vi "test TCX read (installed 71).vi"() -> ()   [LabVIEW 2011] (continued)
nsion/v2\"><Watts>75</Watts></TPX></Extensions></Trackpoint><Trackpoint><Time>2008-03-03T23:08:00Z</Time><Position><LatitudeDegrees>35.861973</LatitudeDegrees><LongitudeDegrees>-78.884526</LongitudeDegrees></Position><AltitudeMeters>78.485</AltitudeMeters><DistanceMeters>12436.936</DistanceMeters><Cadence>73</Cadence><Extensions><TPX xmlns=\"http://www.garmin.com/xmlschemas/ActivityExtension/v2\"><Watts>74</Watts></TPX></Extensions></Trackpoint><Trackpoint><Time>2008-03-03T23:08:01Z</Time><Position><LatitudeDegrees>35.861915</LatitudeDegrees><LongitudeDegrees>-78.884579</LongitudeDegrees></Position><AltitudeMeters>77.523</AltitudeMeters><DistanceMeters>12444.917</DistanceMeters><Cadence>73</Cadence><Extensions><TPX xmlns=\"http://www.garmin.com/xmlschemas/ActivityExtension/v2\"><Watts>81</Watts></TPX></Extensions></Trackpoint><Trackpoint><Time>2008-03-03T23:08:02Z</Time><Position><LatitudeDegrees>35.861859</LatitudeDegrees><LongitudeDegrees>-78.884632</LongitudeDegrees></Position><AltitudeMeters>78.965</AltitudeMeters><DistanceMeters>12452.844</DistanceMeters><Cadence>73</Cadence><Extensions><TPX xmlns=\"http://www.garmin.com/xmlschemas/ActivityExtension/v2\"><Watts>81</Watts></TPX></Extensions></Trackpoint><Trackpoint><Time>2008-03-03T23:08:03Z</Time><Position><LatitudeDegrees>35.861803</LatitudeDegrees><LongitudeDegrees>-78.884687</LongitudeDegrees></Position><AltitudeMeters>78.004</AltitudeMeters><DistanceMeters>12460.762</DistanceMeters><Cadence>73</Cadence><Extensions><TPX xmlns=\"http://www.garmin.com/xmlschemas/ActivityExtension/v2\"><Watts>89</Watts></TPX></Extensions></Trackpoint><Trackpoint><Time>2008-03-03T23:08:04Z</Time><Position><LatitudeDegrees>35.861749</LatitudeDegrees><LongitudeDegrees>-78.884744</LongitudeDegrees></Position><AltitudeMeters>78.004</AltitudeMeters><DistanceMeters>12468.679</DistanceMeters><Cadence>72</Cadence><Extensions><TPX xmlns=\"http://www.garmin.com/xmlschemas/ActivityExtension/v2\"><Watts>91</Watts></TPX></Extensions></Trackpoint><Trackpoint><Time>2008-03-03T23:08:05Z</Time><Position><LatitudeDegrees>35.861695</LatitudeDegrees><LongitudeDegrees>-78.884802</LongitudeDegrees></Position><AltitudeMeters>78.485</AltitudeMeters><DistanceMeters>12476.672</DistanceMeters><Cadence>73</Cadence><Extensions><TPX xmlns=\"http://www.garmin.com/xmlschemas/ActivityExtension/v2\"><Watts>93</Watts></TPX></Extensions></Trackpoint><Trackpoint><Time>2008-03-03T23:08:06Z</Time><Position><LatitudeDegrees>35.861640</LatitudeDegrees><LongitudeDegrees>-78.884862</LongitudeDegrees></Position><AltitudeMeters>77.523</AltitudeMeters><DistanceMeters>12484.829</DistanceMeters><Cadence>75</Cadence><Extensions><TPX xmlns=\"http://www.garmin.com/xmlschemas/ActivityExtension/v2\"><Watts>87</Watts></TPX></Extensions></Trackpoint><Trackpoint><Time>2008-03-03T23:08:07Z</Time><Position><LatitudeDegrees>35.861583</LatitudeDegrees><LongitudeDegrees>-78.884922</LongitudeDegrees></Position><AltitudeMeters>77.043</AltitudeMeters><DistanceMeters>12493.188</DistanceMeters><Cadence>77</Cadence><Extensions><TPX xmlns=\"http://www.garmin.com/xmlschemas/ActivityExtension/v2\"><Watts>79</Watts></TPX></Extensions></Trackpoint><Trackpoint><Time>2008-03-03T23:08:08Z</Time><Position><LatitudeDegrees>35.861522</LatitudeDegrees><LongitudeDegrees>-78.884981</LongitudeDegrees></Position><AltitudeMeters>77.043</AltitudeMeters><DistanceMeters>12501.759</DistanceMeters><Cadence>77</Cadence><Extensions><TPX xmlns=\"http://www.garmin.com/xmlschemas/ActivityExtension/v2\"><Watts>79</Watts></TPX></Extensions></Trackpoint><Trackpoint><Time>2008-03-03T23:08:09Z</Time><Position><LatitudeDegrees>35.861459</LatitudeDegrees><LongitudeDegrees>-78.885040</LongitudeDegrees></Position><AltitudeMeters>77.043</AltitudeMeters><DistanceMeters>12510.541</DistanceMeters><Cadence>75</Cadence><Extensions><TPX xmlns=\"http://www.garmin.com/xmlschemas/ActivityExtension/v2\"><Watts>72</Watts></TPX></Extensions></Trackpoint><Trackpoint><Time>2008-03-03T23:08:10Z</Time><Position><LatitudeDegrees>35.861395</LatitudeDegrees><LongitudeDegrees>-78.885100</LongitudeDegrees></Position><AltitudeMeters>76.562</AltitudeMeters><DistanceMeters>12519.516</DistanceMeters><Cadence>67</Cadence><Extensions><TPX xmlns=\"http://www.garmin.com/xmlschemas/ActivityExtension/v2\"><Watts>71</Watts></TPX></Extensions></Trackpoint><Trackpoint><Time>2008-03-03T23:08:11Z</Time><Position><LatitudeDegrees>35.861330</LatitudeDegrees><LongitudeDegrees>-78.885161</LongitudeDegrees></Position><AltitudeMeters>76.081</AltitudeMeters><DistanceMeters>12528.636</DistanceMeters><Cadence>70</Cadence><Extensions><TPX xmlns=\"http://www.garmin.com/xmlschemas/ActivityExtension/v2\"><Watts>103</Watts></TPX></Extensions></Trackpoint><Trackpoint><Time>2008-03-03T23:08:12Z</Time><Position><LatitudeDegrees>35.861262</LatitudeDegrees><LongitudeDegrees>-78.885224</LongitudeDegrees></Position><AltitudeMeters>76.081</AltitudeMeters><DistanceMeters>12538.094</DistanceMeters><Cadence>70</Cadence><Extensions><TPX xmlns=\"http://www.garmin.com/xmlschemas/ActivityExtension/v2\"><Watts>102</Watts></TPX></Extensions></Trackpoint><Trackpoint><Time>2008-03-03T23:08:13Z</Time><Position><LatitudeDegrees>35.861193</LatitudeDegrees><LongitudeDegrees>-78.885289</LongitudeDegrees></Position><AltitudeMeters>76.081</AltitudeMeters><DistanceMeters>12547.728</DistanceMeters><Cadence>73</Cadence><Extensions><TPX xmlns=\"http://www.garmin.com/xmlschemas/ActivityExtension/v2\"><Watts>136</Watts></TPX></Extensions></Trackpoint><Trackpoint><Time>2008-03-03T23:08:14Z</Time><Position><LatitudeDegrees>35.861124</LatitudeDegrees><LongitudeDegrees>-78.885357</LongitudeDegrees></Position><AltitudeMeters>76.562</AltitudeMeters><DistanceMeters>12557.572</DistanceMeters><Cadence>74</Cadence><Extensions><TPX xmlns=\"http://www.garmin.com/xmlschemas/ActivityExtension/v2\"><Watts>141</Watts></TPX></Extensions></Trackpoint><Trackpoint><Time>2008-03-03T23:08:15Z</Time><Position><LatitudeDegrees>35.861052</LatitudeDegrees><LongitudeDegrees>-78.885425</LongitudeDegrees></Position><AltitudeMeters>75.601</AltitudeMeters><DistanceMeters>12567.610</DistanceMeters><Cadence>76</Cadence><Extensions><TPX xmlns=\"http://www.garmin.com/xmlschemas/ActivityExtension/v2\"><Watts>141</Watts></TPX></Extensions></Trackpoint><Trackpoint><Time>2008-03-03T23:08:16Z</Time><Position><LatitudeDegrees>35.860980</LatitudeDegrees><LongitudeDegrees>-78.885493</LongitudeDegrees></Position><AltitudeMeters>76.081</AltitudeMeters><DistanceMeters>12577.708</DistanceMeters><Cadence>76</Cadence><Extensions><TPX xmlns=\"http://www.garmin.com/xmlschemas/ActivityExtension/v2\"><Watts>124</Watts></TPX></Extensions></Trackpoint><Trackpoint><Time>2008-03-03T23:08:17Z</Time><Position><LatitudeDegrees>35.860907</LatitudeDegrees><LongitudeDegrees>-78.885559</LongitudeDegrees></Position><AltitudeMeters>75.601</AltitudeMeters><DistanceMeters>12587.827</DistanceMeters><Cadence>76</Cadence><Extensions><TPX xmlns=\"http://www.garmin.com/xmlschemas/ActivityExtension/v2\"><Watts>107</Watts></TPX></Extensions></Trackpoint><Trackpoint><Time>2008-03-03T23:08:18Z</Time><Position><LatitudeDegrees>35.860833</LatitudeDegrees><LongitudeDegrees>-78.885625</LongitudeDegrees></Position><AltitudeMeters>75.120</AltitudeMeters><DistanceMeters>12597.975</DistanceMeters><Cadence>77</Cadence><Extensions><TPX xmlns=\"http://www.garmin.com/xmlschemas/ActivityExtension/v2\"><Watts>106</Watts></TPX></Extensions></Trackpoint><Trackpoint><Time>2008-03-03T23:08:19Z</Time><Position><LatitudeDegrees>35.860758</LatitudeDegrees><LongitudeDegrees>-78.885691</LongitudeDegrees></Position><AltitudeMeters>76.081</AltitudeMeters><DistanceMeters>12608.146</DistanceMeters><Cadence>77</Cadence><Extensions><TPX xmlns=\"http://www.garmin.com/xmlschemas/ActivityExtension/v2\"><Watts>100</Watts></TPX></Extensions></Trackpoint><Trackpoint><Time>2008-03-03T23:08:20Z</Time><Position><LatitudeDegrees>35.860684</LatitudeDegrees><LongitudeDegrees>-78.885756</LongitudeDegrees></Position><AltitudeMeters>75.120</AltitudeMeters><DistanceMeters>12618.253</DistanceMeters><Cadence>76</Cadence><Extensions><TPX xmlns=\"http://www.garmin.com/xmlschemas/ActivityExtension/v2\"><Watts>97</Watts></TPX></Extensions></Trackpoint><Trackpoint><Time>2008-03-03T23:08:21Z</Time><Position><LatitudeDegrees>35.860610</LatitudeDegrees><LongitudeDegrees>-78.885821</LongitudeDegrees></Position><AltitudeMeters>74.640</AltitudeMeters><DistanceMeters>12628.325</DistanceMeters><Cadence>76</Cadence><Extensions><TPX xmlns=\"http://www.garmin.com/xmlschemas/ActivityExtension/v2\"><Watts>101</Watts></TPX></Extensions></Trackpoint><Trackpoint><Time>2008-03-03T23:08:22Z</Time><Position><LatitudeDegrees>35.860538</LatitudeDegrees><LongitudeDegrees>-78.885887</LongitudeDegrees></Position><AltitudeMeters>75.120</AltitudeMeters><DistanceMeters>12638.349</DistanceMeters><Cadence>76</Cadence><Extensions><TPX xmlns=\"http://www.garmin.com/xmlschemas/ActivityExtension/v2\"><Watts>94</Watts></TPX></Extensions></Trackpoint><Trackpoint><Time>2008-03-03T23:08:23Z</Time><Position><LatitudeDegrees>35.860466</LatitudeDegrees><LongitudeDegrees>-78.885953</LongitudeDegrees></Position><AltitudeMeters>74.640</AltitudeMeters><DistanceMeters>12648.291</DistanceMeters><Cadence>75</Cadence><Extensions><TPX xmlns=\"http://www.garmin.com/xmlschemas/ActivityExtension/v2\"><Watts>98</Watts></TPX></Extensions></Trackpoint><Trackpoint><Time>2008-03-03T23:08:24Z</Time><Position><LatitudeDegrees>35.860393</LatitudeDegrees><LongitudeDegrees>-78.886017</LongitudeDegrees></Position><AltitudeMeters>74.640</AltitudeMeters><DistanceMeters>12658.178</DistanceMeters><Cadence>75</Cadence><Extensions><TPX xmlns=\"http://www.garmin.com/xmlschemas/ActivityExtension/v2\"><Watts>92</Watts></TPX></Extensions></Trackpoint><Trackpoint><Time>2008-03-03T23:08:25Z</Time><Position><LatitudeDegrees>35.860320</LatitudeDegrees><LongitudeDegrees>-78.886080</LongitudeDegrees></Position><AltitudeMeters>74.159</AltitudeMeters><DistanceMeters>12668.053</DistanceMeters><Cadence>74</Cadence><Extensions><TPX xmlns=\"http://www.garmin.com/xmlschemas/ActivityExtension/v2\"><Watts>62</Watts></TPX></Extensions></Trackpoint><Trackpoint><Time>2008-03-03T23:08:26Z</Time><Position><LatitudeDegrees>35.860248</LatitudeDegrees><LongitudeDegrees>-78.886143</LongitudeDegrees></Position><AltitudeMeters>74.159</AltitudeMeters><DistanceMeters>12677.914</DistanceMeters><Cadence>74</Cadence><Extensions><TPX xmlns=\"http://www.garmin.com/xmlschemas/ActivityExtension/v2\"><Watts>62</Watts></TPX></Extensions></Trackpoint><Trackpoint><Time>2008-03-03T23:08:27Z</Time><Position><LatitudeDegrees>35.860178</LatitudeDegrees><LongitudeDegrees>-78.886208</LongitudeDegrees></Position><AltitudeMeters>74.159</AltitudeMeters><DistanceMeters>12687.683</DistanceMeters><Cadence>0</Cadence></Trackpoint><Trackpoint><Time>2008-03-03T23:08:28Z</Time><Position><LatitudeDegrees>35.860108</LatitudeDegrees><LongitudeDegrees>-78.886273</LongitudeDegrees></Position><AltitudeMeters>73.678</AltitudeMeters><DistanceMeters>12697.343</DistanceMeters><Cadence>0</Cadence></Trackpoint><Trackpoint><Time>2008-03-03T23:08:29Z</Time><Position><LatitudeDegrees>35.860044</LatitudeDegrees><LongitudeDegrees>-78.886338</LongitudeDegrees></Position><AltitudeMeters>73.198</AltitudeMeters><DistanceMeters>12706.586</DistanceMeters><Cadence>0</Cadence></Trackpoint><Trackpoint><Time>2008-03-03T23:08:30Z</Time><Position><LatitudeDegrees>35.859989</LatitudeDegrees><LongitudeDegrees>-78.886398</LongitudeDegrees></Position><AltitudeMeters>72.236</AltitudeMeters><DistanceMeters>12714.678</DistanceMeters><Cadence>12</Cadence></Trackpoint><Trackpoint><Time>2008-03-03T23:08:31Z</Time><Position><LatitudeDegrees>35.859945</LatitudeDegrees><LongitudeDegrees>-78.886452</LongitudeDegrees></Position><AltitudeMeters>72.236</AltitudeMeters><DistanceMeters>12721.393</DistanceMeters><Cadence>12</Cadence></Trackpoint><Trackpoint><Time>2008-03-03T23:08:32Z</Time><Position><LatitudeDegrees>35.859913</LatitudeDegrees><LongitudeDegrees>-78.886498</LongitudeDegrees></Position><AltitudeMeters>72.236</AltitudeMeters><DistanceMeters>12726.843</DistanceMeters><Cadence>0</Cadence></Trackpoint><Trackpoint><Time>2008-03-03T23:08:33Z</Time><Position><LatitudeDegrees>35.859889</LatitudeDegrees><LongitudeDegrees>-78.886536</LongitudeDegrees></Position><AltitudeMeters>72.236</AltitudeMeters><DistanceMeters>12731.098</DistanceMeters><Cadence>0</Cadence></Trackpoint><Trackpoint><Time>2008-03-03T23:08:34Z</Time><Position><LatitudeDegrees>35.859876</LatitudeDegrees><LongitudeDegrees>-78.886567</LongitudeDegrees></Position><AltitudeMeters>71.755</AltitudeMeters><DistanceMeters>12734.231</DistanceMeters><Cadence>18</Cadence></Trackpoint><Trackpoint><Time>2008-03-03T23:08:35Z</Time><Position><LatitudeDegrees>35.859867</LatitudeDegrees><LongitudeDegrees>-78.886602</LongitudeDegrees></Position><AltitudeMeters>71.755</AltitudeMeters><DistanceMeters>12737.604</DistanceMeters><Cadence>34</Cadence><Extensions><TPX xmlns=\"http://www.garmin.com/xmlschemas/ActivityExtension/v2\"><Watts>182</Watts></TPX></Extensions></Trackpoint><Trackpoint><Time>2008-03-03T23:08:36Z</Time><Position><LatitudeDegrees>35.859866</LatitudeDegrees><LongitudeDegrees>-78.886648</LongitudeDegrees></Position><AltitudeMeters>71.755</AltitudeMeters><DistanceMeters>12741.797</DistanceMeters><Cadence>34</Cadence><Extensions><TPX xmlns=\"http://www.garmin.com/xmlschemas/ActivityExtension/v2\"><Watts>179</Watts></TPX></Extensions></Trackpoint><Trackpoint><Time>2008-03-03T23:08:37Z</Time><Position><LatitudeDegrees>35.859876</LatitudeDegrees><LongitudeDegrees>-78.886705</LongitudeDegrees></Position><AltitudeMeters>71.755</AltitudeMeters><DistanceMeters>12747.175</DistanceMeters><Cadence>49</Cadence><Extensions><TPX xmlns=\"http://www.garmin.com/xmlschemas/ActivityExtension/v2\"><Watts>302</Watts></TPX></Extensions></Trackpoint><Trackpoint><Time>2008-03-03T23:08:38Z</Time><Position><LatitudeDegrees>35.859892</LatitudeDegrees><LongitudeDegrees>-78.886772</LongitudeDegrees></Position><AltitudeMeters>71.755</AltitudeMeters><DistanceMeters>12753.439</DistanceMeters><Cadence>58</Cadence><Extensions><TPX xmlns=\"http://www.garmin.com/xmlschemas/ActivityExtension/v2\"><Watts>428</Watts></TPX></Extensions></Trackpoint><Trackpoint><Time>2008-03-03T23:08:39Z</Time><Position><LatitudeDegrees>35.859909</LatitudeDegrees><LongitudeDegrees>-78.886846</LongitudeDegrees></Position><AltitudeMeters>71.755</AltitudeMeters><DistanceMeters>12760.476</DistanceMeters><Cadence>58</Cadence><Extensions><TPX xmlns=\"http://www.garmin.com/xmlschemas/ActivityExtension/v2\"><Watts>428</Watts></TPX></Extensions></Trackpoint><Trackpoint><Time>2008-03-03T23:08:40Z</Time><Position><LatitudeDegrees>35.859929</LatitudeDegrees><LongitudeDegrees>-78.886927</LongitudeDegrees></Position><AltitudeMeters>71.755</AltitudeMeters><DistanceMeters>12768.110</DistanceMeters><Cadence>74</Cadence><Extensions><TPX xmlns=\"http://www.garmin.com/xmlschemas/ActivityExtension/v2\"><Watts>465</Watts></TPX></Extensions></Trackpoint><Trackpoint><Time>2008-03-03T23:08:41Z</Time><Position><LatitudeDegrees>35.859949</LatitudeDegrees><LongitudeDegrees>-78.887013</LongitudeDegrees></Position><AltitudeMeters>72.236</AltitudeMeters><DistanceMeters>12776.246</DistanceMeters><Cadence>74</Cadence><Extensions><TPX xmlns=\"http://www.garmin.com/xmlschemas/ActivityExtension/v2\"><Watts>470</Watts></TPX></Extensions></Trackpoint><Trackpoint><Time>2008-03-03T23:08:42Z</Time><Position><LatitudeDegrees>35.859970</LatitudeDegrees><LongitudeDegrees>-78.887104</LongitudeDegrees></Position><AltitudeMeters>72.236</AltitudeMeters><DistanceMeters>12784.849</DistanceMeters><Cadence>79</Cadence><Extensions><TPX xmlns=\"http://www.garmin.com/xmlschemas/ActivityExtension/v2\"><Watts>395</Watts></TPX></Extensions></Trackpoint><Trackpoint><Time>2008-03-03T23:08:43Z</Time><Position><LatitudeDegrees>35.859993</LatitudeDegrees><LongitudeDegrees>-78.887199</LongitudeDegrees></Position><AltitudeMeters>72.236</AltitudeMeters><DistanceMeters>12793.792</DistanceMeters><Cadence>85</Cadence><Extensions><TPX xmlns=\"http://www.garmin.com/xmlschemas/ActivityExtension/v2\"><Watts>366</Watts></TPX></Extensions></Trackpoint><Trackpoint><Time>2008-03-03T23:08:44Z</Time><Position><LatitudeDegrees>35.860014</LatitudeDegrees><LongitudeDegrees>-78.887299</LongitudeDegrees></Position><AltitudeMeters>72.236</AltitudeMeters><DistanceMeters>12803.111</DistanceMeters><Cadence>87</Cadence><Extensions><TPX xmlns=\"http://www.garmin.com/xmlschemas/ActivityExtension/v2\"><Watts>420</Watts></TPX></Extensions></Trackpoint><Trackpoint><Time>2008-03-03T23:08:45Z</Time><Position><LatitudeDegrees>35.860035</LatitudeDegrees><LongitudeDegrees>-78.887402</LongitudeDegrees></Position><AltitudeMeters>72.717</AltitudeMeters><DistanceMeters>12812.741</DistanceMeters><Cadence>91</Cadence><Extensions><TPX xmlns=\"http://www.garmin.com/xmlschemas/ActivityExtension/v2\"><Watts>485</Watts></TPX></Extensions></Trackpoint><Trackpoint><Time>2008-03-03T23:08:46Z</Time><Position><LatitudeDegrees>35.860057</LatitudeDegrees><LongitudeDegrees>-78.887508</LongitudeDegrees></Position><AltitudeMeters>72.717</AltitudeMeters><DistanceMeters>12822.614</DistanceMeters><Cadence>92</Cadence><Extensions><TPX xmlns=\"http://www.garmin.com/xmlschemas/ActivityExtension/v2\"><Watts>483</Watts></TPX></Extensions></Trackpoint><Trackpoint><Time>2008-03-03T23:08:47Z</Time><Position><LatitudeDegrees>35.860078</LatitudeDegrees><LongitudeDegrees>-78.887616</LongitudeDegrees></Position><AltitudeMeters>73.678</AltitudeMeters><DistanceMeters>12832.634</DistanceMeters><Cadence>93</Cadence><Extensions><TPX xmlns=\"http://www.garmin.com/xmlschemas/ActivityExtension/v2\"><Watts>477</Watts></TPX></Extensions></Trackpoint><Trackpoint><Time>2008-03-03T23:08:48Z</Time><Position><LatitudeDegrees>35.860097</LatitudeDegrees><LongitudeDegrees>-78.887724</LongitudeDegrees></Position><AltitudeMeters>73.198</AltitudeMeters><DistanceMeters>12842.673</DistanceMeters><Cadence>93</Cadence><Extensions><TPX xmlns=\"http://www.garmin.com/xmlschemas/ActivityExtension/v2\"><Watts>388</Watts></TPX></Extensions></Trackpoint><Trackpoint><Time>2008-03-03T23:08:49Z</Time><Position><LatitudeDegrees>35.860116</LatitudeDegrees><LongitudeDegrees>-78.887833</LongitudeDegrees></Position><AltitudeMeters>73.198</AltitudeMeters><DistanceMeters>12852.671</DistanceMeters><Cadence>92</Cadence><Extensions><TPX xmlns=\"http://www.garmin.com/xmlschemas/ActivityExtension/v2\"><Watts>266</Watts></TPX></Extensions></Trackpoint><Trackpoint><Time>2008-03-03T23:08:50Z</Time><Position><LatitudeDegrees>35.860134</LatitudeDegrees><LongitudeDegrees>-78.887941</LongitudeDegrees></Position><AltitudeMeters>73.678</AltitudeMeters><DistanceMeters>12862.609</DistanceMeters><Cadence>91</Cadence><Extensions><TPX xmlns=\"http://www.garmin.com/xmlschemas/ActivityExtension/v2\"><Watts>169</Watts></TPX></Extensions></Trackpoint><Trackpoint><Time>2008-03-03T23:08:51Z</Time><Position><LatitudeDegrees>35.860150</LatitudeDegrees><LongitudeDegrees>-78.888048</LongitudeDegrees></Position><AltitudeMeters>73.678</AltitudeMeters><DistanceMeters>12872.501</DistanceMeters><Cadence>91</Cadence><Extensions><TPX xmlns=\"http://www.garmin.com/xmlschemas/ActivityExtension/v2\"><Watts>169</Watts></TPX></Extensions></Trackpoint><Trackpoint><Time>2008-03-03T23:08:52Z</Time><Position><LatitudeDegrees>35.860166</LatitudeDegrees><LongitudeDegrees>-78.888155</LongitudeDegrees></Position><AltitudeMeters>73.678</AltitudeMeters><DistanceMeters>12882.326</DistanceMeters><Cadence>90</Cadence><Extensions><TPX xmlns=\"http://www.garmin.com/xmlschemas/ActivityExtension/v2\"><Watts>150</Watts></TPX></Extensions></Trackpoint><Trackpoint><Time>2008-03-03T23:08:53Z</Time><Position><LatitudeDegrees>35.860180</LatitudeDegrees><LongitudeDegrees>-78.888263</LongitudeDegrees></Position><AltitudeMeters>73.198</AltitudeMeters><DistanceMeters>12892.139</DistanceMeters><Cadence>91</Cadence><Extensions><TPX xmlns=\"http://www.garmin.com/xmlschemas/ActivityExtension/v2\"><Watts>136</Watts></TPX></Extensions></Trackpoint><Trackpoint><Time>2008-03-03T23:08:54Z</Time><Position><LatitudeDegrees>35.860195</LatitudeDegrees><LongitudeDegrees>-78.888370</LongitudeDegrees></Position><AltitudeMeters>73.198</AltitudeMeters><DistanceMeters>12901.978</DistanceMeters><Cadence>80</Cadence><Extensions><TPX xmlns=\"http://www.garmin.com/xmlschemas/ActivityExtension/v2\"><Watts>121</Watts></TPX></Extensions></Trackpoint><Trackpoint><Time>2008-03-03T23:08:55Z</Time><Position><LatitudeDegrees>35.860208</LatitudeDegrees><LongitudeDegrees>-78.888479</LongitudeDegrees></Position><AltitudeMeters>73.678</AltitudeMeters><DistanceMeters>12911.919</DistanceMeters><Cadence>81</Cadence><Extensions><TPX xmlns=\"http://www.garmin.com/xmlschemas/ActivityExtension/v2\"><Watts>113</Watts></TPX></Extensions></Trackpoint><Trackpoint><Time>2008-03-03T23:08:56Z</Time><Position><LatitudeDegrees>35.860222</LatitudeDegrees><LongitudeDegrees>-78.888589</LongitudeDegrees></Position><AltitudeMeters>72.717</AltitudeMeters><DistanceMeters>12921.953</DistanceMeters><Cadence>82</Cadence><Extensions><TPX xmlns=\"http://www.garmin.com/xmlschemas/ActivityExtension/v2\"><Watts>115</Watts></TPX></Extensions></Trackpoint><Trackpoint><Time>2008-03-03T23:08:57Z</Time><Position><LatitudeDegrees>35.860233</LatitudeDegrees><LongitudeDegrees>-78.888701</LongitudeDegrees></Position><AltitudeMeters>72.717</AltitudeMeters><DistanceMeters>12932.187</DistanceMeters><Cadence>83</Cadence><Extensions><TPX xmlns=\"http://www.garmin.com/xmlschemas/ActivityExtension/v2\"><Watts>113</Watts></TPX></Extensions></Trackpoint><Trackpoint><Time>2008-03-03T23:08:58Z</Time><Position><LatitudeDegrees>35.860244</LatitudeDegrees><LongitudeDegrees>-78.888815</LongitudeDegrees></Position><AltitudeMeters>72.717</AltitudeMeters><DistanceMeters>12942.533</DistanceMeters><Cadence>86</Cadence><Extensions><TPX xmlns=\"http://www.garmin.com/xmlschemas/ActivityExtension/v2\"><Watts>81</Watts></TPX></Extensions></Trackpoint><Trackpoint><Time>2008-03-03T23:08:59Z</Time><Position><LatitudeDegrees>35.860255</LatitudeDegrees><LongitudeDegrees>-78.888931</LongitudeDegrees></Position><AltitudeMeters>72.236</AltitudeMeters><DistanceMeters>12953.332</DistanceMeters><Cadence>86</Cadence><Extensions><TPX xmlns=\"http://www.garmin.com/xmlschemas/ActivityExtension/v2\"><Watts>80</Watts></TPX></Extensions></Trackpoint><Trackpoint><Time>2008-03-03T23:09:00Z</Time><Position><LatitudeDegrees>35.860269</LatitudeDegrees><LongitudeDegrees>-78.889050</LongitudeDegrees></Position><AltitudeMeters>72.236</AltitudeMeters><DistanceMeters>12964.036</DistanceMeters><Cadence>89</Cadence><Extensions><TPX xmlns=\"http://www.garmin.com/xmlschemas/ActivityExtension/v2\"><Watts>84</Watts></TPX></Extensions></Trackpoint><Trackpoint><Time>2008-03-03T23:09:01Z</Time><Position><LatitudeDegrees>35.860285</LatitudeDegrees><LongitudeDegrees>-78.889171</LongitudeDegrees></Position><AltitudeMeters>71.755</AltitudeMeters><DistanceMeters>12975.059</DistanceMeters><Cadence>89</Cadence><Extensions><TPX xmlns=\"http://www.garmin.com/xmlschemas/ActivityExtension/v2\"><Watts>90</Watts></TPX></Extensions></Trackpoint><Trackpoint><Time>2008-03-03T23:09:02Z</Time><Position><LatitudeDegrees>35.860300</LatitudeDegrees><LongitudeDegrees>-78.889294</LongitudeDegrees></Position><AltitudeMeters>71.755</AltitudeMeters><DistanceMeters>12986.354</DistanceMeters><Cadence>87</Cadence><Extensions><TPX xmlns=\"http://www.garmin.com/xmlschemas/ActivityExtension/v2\"><Watts>115</Watts></TPX></Extensions></Trackpoint><Trackpoint><Time>2008-03-03T23:09:03Z</Time><Position><LatitudeDegrees>35.860315</LatitudeDegrees><LongitudeDegrees>-78.889421</LongitudeDegrees></Position><AltitudeMeters>71.275</AltitudeMeters><DistanceMeters>12997.958</DistanceMeters><Cadence>89</Cadence><Extensions><TPX xmlns=\"http://www.garmin.com/xmlschemas/ActivityExtension/v2\"><Watts>147</Watts></TPX></Extensions></Trackpoint><Trackpoint><Time>2008-03-03T23:09:04Z</Time><Position><LatitudeDegrees>35.860331</LatitudeDegrees><LongitudeDegrees>-78.889552</LongitudeDegrees></Position><AltitudeMeters>71.275</AltitudeMeters><DistanceMeters>13009.899</DistanceMeters><Cadence>92</Cadence><Extensions><TPX xmlns=\"http://www.garmin.com/xmlschemas/ActivityExtension/v2\"><Watts>145</Watts></TPX></Extensions></Trackpoint><Trackpoint><Time>2008-03-03T23:09:05Z</Time><Position><LatitudeDegrees>35.860348</LatitudeDegrees><LongitudeDegrees>-78.889685</LongitudeDegrees></Position><AltitudeMeters>70.794</AltitudeMeters><DistanceMeters>13022.080</DistanceMeters><Cadence>94</Cadence><Extensions><TPX xmlns=\"http://www.garmin.com/xmlschemas/ActivityExtension/v2\"><Watts>146</Watts></TPX></Extensions></Trackpoint><Trackpoint><Time>2008-03-03T23:09:06Z</Time><Position><LatitudeDegrees>35.860365</LatitudeDegrees><LongitudeDegrees>-78.889821</LongitudeDegrees></Position><AltitudeMeters>70.313</AltitudeMeters><DistanceMeters>13034.580</DistanceMeters><Cadence>94</Cadence><Extensions><TPX xmlns=\"http://www.garmin.com/xmlschemas/ActivityExtension/v2\"><Watts>145</Watts></TPX></Extensions></Trackpoint><Trackpoint><Time>2008-03-03T23:09:07Z</Time><Position><LatitudeDegrees>35.860383</LatitudeDegrees><LongitudeDegrees>-78.889961</LongitudeDegrees></Position><AltitudeMeters>70.313</AltitudeMeters><DistanceMeters>13047.376</DistanceMeters><Cadence>90</Cadence><Extensions><TPX xmlns=\"http://www.garmin.com/xmlschemas/ActivityExtension/v2\"><Watts>128</Watts></TPX></Extensions></Trackpoint><Trackpoint><Time>2008-03-03T23:09:08Z</Time><Position><LatitudeDegrees>35.860400</LatitudeDegrees><LongitudeDegrees>-78.890102</LongitudeDegrees></Position><AltitudeMeters>69.833</AltitudeMeters><DistanceMeters>13060.242</DistanceMeters><Cadence>92</Cadence><Extensions><TPX xmlns=\"http://www.garmin.com/xmlschemas/ActivityExtension/v2\"><Watts>125</Watts></TPX></Extensions></Trackpoint><Trackpoint><Time>2008-03-03T23:09:09Z</Time><Position><LatitudeDegrees>35.860418</LatitudeDegrees><LongitudeDegrees>-78.890245</LongitudeDegrees></Position><AltitudeMeters>69.833</AltitudeMeters><DistanceMeters>13073.274</DistanceMeters><Cadence>92</Cadence><Extensions><TPX xmlns=\"http://www.garmin.com/xmlschemas/ActivityExtension/v2\"><Watts>112</Watts></TPX></Extensions></Trackpoint><Trackpoint><Time>2008-03-03T23:09:10Z</Time><Position><LatitudeDegrees>35.860435</LatitudeDegrees><LongitudeDegrees>-78.890388</LongitudeDegrees></Position><AltitudeMeters>69.833</AltitudeMeters><DistanceMeters>13086.366</DistanceMeters><Cadence>92</Cadence><Extensions><TPX xmlns=\"http://www.garmin.com/xmlschemas/ActivityExtension/v2\"><Watts>95</Watts></TPX></Extensions></Trackpoint><Trackpoint><Time>2008-03-03T23:09:11Z</Time><Position><LatitudeDegrees>35.860454</LatitudeDegrees><LongitudeDegrees>-78.890529</LongitudeDegrees></Position><AltitudeMeters>69.352</AltitudeMeters><DistanceMeters>13099.340</DistanceMeters><Cadence>92</Cadence><Extensions><TPX xmlns=\"http://www.garmin.com/xmlschemas/ActivityExtension/v2\"><Watts>96</Watts></TPX></Extensions></Trackpoint><Trackpoint><Time>2008-03-03T23:09:12Z</Time><Position><LatitudeDegrees>35.860473</LatitudeDegrees><LongitudeDegrees>-78.890670</LongitudeDegrees></Position><AltitudeMeters>69.352</AltitudeMeters><DistanceMeters>13112.229</DistanceMeters><Cadence>90</Cadence><Extensions><TPX xmlns=\"http://www.garmin.com/xmlschemas/ActivityExtension/v2\"><Watts>85</Watts></TPX></Extensions></Trackpoint><Trackpoint><Time>2008-03-03T23:09:13Z</Time><Position><LatitudeDegrees>35.860491</LatitudeDegrees><LongitudeDegrees>-78.890808</LongitudeDegrees></Position><AltitudeMeters>68.872</AltitudeMeters><DistanceMeters>13124.790</DistanceMeters><Cadence>89</Cadence><Extensions><TPX xmlns=\"http://www.garmin.com/xmlschemas/ActivityExtension/v2\"><Watts>79</Watts></TPX></Extensions></Trackpoint><Trackpoint><Time>2008-03-03T23:09:14Z</Time><Position><LatitudeDegrees>35.860509</LatitudeDegrees><LongitudeDegrees>-78.890945</LongitudeDegrees></Position><AltitudeMeters>68.391</AltitudeMeters><DistanceMeters>13137.343</DistanceMeters><Cadence>88</Cadence><Extensions><TPX xmlns=\"http://www.garmin.com/xmlschemas/ActivityExtension/v2\"><Watts>80</Watts></TPX></Extensions></Trackpoint><Trackpoint><Time>2008-03-03T23:09:15Z</Time><Position><LatitudeDegrees>35.860528</LatitudeDegrees><LongitudeDegrees>-78.891081</LongitudeDegrees></Position><AltitudeMeters>68.391</AltitudeMeters><DistanceMeters>13149.784</DistanceMeters><Cadence>88</Cadence><Extensions><TPX xmlns=\"http://www.garmin.com/xmlschemas/ActivityExtension/v2\"><Watts>84</Watts></TPX></Extensions></Trackpoint><Trackpoint><Time>2008-03-03T23:09:16Z</Time><Position><LatitudeDegrees>35.860547</LatitudeDegrees><LongitudeDegrees>-78.891217</LongitudeDegrees></Position><AltitudeMeters>68.872</AltitudeMeters><DistanceMeters>13162.190</DistanceMeters><Cadence>88</Cadence><Extensions><TPX xmlns=\"http://www.garmin.com/xmlschemas/ActivityExtension/v2\"><Watts>84</Watts></TPX></Extensions></Trackpoint><Trackpoint><Time>2008-03-03T23:09:17Z</Time><Position><LatitudeDegrees>35.860567</LatitudeDegrees><LongitudeDegrees>-78.891351</LongitudeDegrees></Position><AltitudeMeters>68.391</AltitudeMeters><DistanceMeters>13174.573</DistanceMeters><Cadence>87</Cadence><Extensions><TPX xmlns=\"http://www.garmin.com/xmlschemas/ActivityExtension/v2\"><Watts>90</Watts></TPX></Extensions></Trackpoint><Trackpoint><Time>2008-03-03T23:09:18Z</Time><Position><LatitudeDegrees>35.860588</LatitudeDegrees><LongitudeDegrees>-78.891485</LongitudeDegrees></Position><AltitudeMeters>67.910</AltitudeMeters><DistanceMeters>13186.806</DistanceMeters><Cadence>87</Cadence><Extensions><TPX xmlns=\"http://www.garmin.com/xmlschemas/ActivityExtension/v2\"><Watts>94</Watts></TPX></Extensions></Trackpoint><Trackpoint><Time>2008-03-03T23:09:19Z</Time><Position><LatitudeDegrees>35.860608</LatitudeDegrees><LongitudeDegrees>-78.891618</LongitudeDegrees></Position><AltitudeMeters>67.910</AltitudeMeters><DistanceMeters>13199.102</DistanceMeters><Cadence>86</Cadence><Extensions><TPX xmlns=\"http://www.garmin.com/xmlschemas/ActivityExtension/v2\"><Watts>108</Watts></TPX></Extensions></Trackpoint><Trackpoint><Time>2008-03-03T23:09:20Z</Time><Position><LatitudeDegrees>35.860630</LatitudeDegrees><LongitudeDegrees>-78.891751</LongitudeDegrees></Position><AltitudeMeters>67.430</AltitudeMeters><DistanceMeters>13211.372</DistanceMeters><Cadence>86</Cadence><Extensions><TPX xmlns=\"http://www.garmin.com/xmlschemas/ActivityExtension/v2\"><Watts>95</Watts></TPX></Extensions></Trackpoint><Trackpoint><Time>2008-03-03T23:09:21Z</Time><Position><LatitudeDegrees>35.860650</LatitudeDegrees><LongitudeDegrees>-78.891884</LongitudeDegrees></Position><AltitudeMeters>67.430</AltitudeMeters><DistanceMeters>13223.512</DistanceMeters><Cadence>86</Cadence><Extensions><TPX xmlns=\"http://www.garmin.com/xmlschemas/ActivityExtension/v2\"><Watts>95</Watts></TPX></Extensions></Trackpoint><Trackpoint><Time>2008-03-03T23:09:22Z</Time><Position><LatitudeDegrees>35.860670</LatitudeDegrees><LongitudeDegrees>-78.892015</LongitudeDegrees></Position><AltitudeMeters>67.430</AltitudeMeters><DistanceMeters>13235.623</DistanceMeters><Cadence>85</Cadence><Extensions><TPX xmlns=\"http://www.garmin.com/xmlschemas/ActivityExtension/v2\"><Watts>90</Watts></TPX></Extensions></Trackpoint><Trackpoint><Time>2008-03-03T23:09:23Z</Time><Position><LatitudeDegrees>35.860690</LatitudeDegrees><LongitudeDegrees>-78.892147</LongitudeDegrees></Position><AltitudeMeters>66.468</AltitudeMeters><DistanceMeters>13247.687</DistanceMeters><Cadence>85</Cadence><Extensions><TPX xmlns=\"http://www.garmin.com/xmlschemas/ActivityExtension/v2\"><Watts>105</Watts></TPX></Extensions></Trackpoint><Trackpoint><Time>2008-03-03T23:09:24Z</Time><Position><LatitudeDegrees>35.860710</LatitudeDegrees><LongitudeDegrees>-78.892277</LongitudeDegrees></Position><AltitudeMeters>66.949</AltitudeMeters><DistanceMeters>13259.637</DistanceMeters><Cadence>84</Cadence><Extensions><TPX xmlns=\"http://www.garmin.com/xmlschemas/ActivityExtension/v2\"><Watts>105</Watts></TPX></Extensions></Trackpoint><Trackpoint><Time>2008-03-03T23:09:25Z</Time><Position><LatitudeDegrees>35.860729</LatitudeDegrees><LongitudeDegrees>-78.892406</LongitudeDegrees></Position><AltitudeMeters>67.430</AltitudeMeters><DistanceMeters>13271.526</DistanceMeters><Cadence>83</Cadence><Extensions><TPX xmlns=\"http://www.garmin.com/xmlschemas/ActivityExtension/v2\"><Watts>84</Watts></TPX></Extensions></Trackpoint><Trackpoint><Time>2008-03-03T23:09:26Z</Time><Position><LatitudeDegrees>35.860747</LatitudeDegrees><LongitudeDegrees>-78.892535</LongitudeDegrees></Position><AltitudeMeters>66.468</AltitudeMeters><DistanceMeters>13283.274</DistanceMeters><Cadence>83</Cadence><Extensions><TPX xmlns=\"http://www.garmin.com/xmlschemas/ActivityExtension/v2\"><Watts>84</Watts></TPX></Extensions></Trackpoint><Trackpoint><Time>2008-03-03T23:09:27Z</Time><Position><LatitudeDegrees>35.860764</LatitudeDegrees><LongitudeDegrees>-78.892661</LongitudeDegrees></Position><AltitudeMeters>66.468</AltitudeMeters><DistanceMeters>13294.882</DistanceMeters><Cadence>81</Cadence><Extensions><TPX xmlns=\"http://www.garmin.com/xmlschemas/ActivityExtension/v2\"><Watts>78</Watts></TPX></Extensions></Trackpoint><Trackpoint><Time>2008-03-03T23:09:28Z</Time><Position><LatitudeDegrees>35.860782</LatitudeDegrees><LongitudeDegrees>-78.892787</LongitudeDegrees></Position><AltitudeMeters>66.949</AltitudeMeters><DistanceMeters>13306.379</DistanceMeters><Cadence>81</Cadence><Extensions><TPX xmlns=\"http://www.garmin.com/xmlschemas/ActivityExtension/v2\"><Watts>94</Watts></TPX></Extensions></Trackpoint><Trackpoint><Time>2008-03-03T23:09:29Z</Time><Position><LatitudeDegrees>35.860800</LatitudeDegrees><LongitudeDegrees>-78.892914</LongitudeDegrees></Position><AltitudeMeters>65.026</AltitudeMeters><DistanceMeters>13318.007</DistanceMeters><Cadence>82</Cadence><Extensions><TPX xmlns=\"http://www.garmin.com/xmlschemas/ActivityExtension/v2\"><Watts>111</Watts></TPX></Extensions></Trackpoint><Trackpoint><Time>2008-03-03T23:09:30Z</Time><Position><LatitudeDegrees>35.860816</LatitudeDegrees><LongitudeDegrees>-78.893044</LongitudeDegrees></Position><AltitudeMeters>64.546</AltitudeMeters><DistanceMeters>13329.932</DistanceMeters><Cadence>84</Cadence><Extensions><TPX xmlns=\"http://www.garmin.com/xmlschemas/ActivityExtension/v2\"><Watts>125</Watts></TPX></Extensions></Trackpoint><Trackpoint><Time>2008-03-03T23:09:31Z</Time><Position><LatitudeDegrees>35.860832</LatitudeDegrees><LongitudeDegrees>-78.893178</LongitudeDegrees></Position><AltitudeMeters>65.026</AltitudeMeters><DistanceMeters>13342.206</DistanceMeters><Cadence>87</Cadence><Extensions><TPX xmlns=\"http://www.garmin.com/xmlschemas/ActivityExtension/v2\"><Watts>125</Watts></TPX></Extensions></Trackpoint><Trackpoint><Time>2008-03-03T23:09:32Z</Time><Position><LatitudeDegrees>35.860851</LatitudeDegrees><LongitudeDegrees>-78.893316</LongitudeDegrees></Position><AltitudeMeters>64.065</AltitudeMeters><DistanceMeters>13354.903</DistanceMeters><Cadence>90</Cadence><Extensions><TPX xmlns=\"http://www.garmin.com/xmlschemas/ActivityExtension/v2\"><Watts>112</Watts></TPX></Extensions></Trackpoint><Trackpoint><Time>2008-03-03T23:09:33Z</Time><Position><LatitudeDegrees>35.860872</LatitudeDegrees><LongitudeDegrees>-78.893458</LongitudeDegrees></Position><AltitudeMeters>63.584</AltitudeMeters><DistanceMeters>13367.898</DistanceMeters><Cadence>93</Cadence><Extensions><TPX xmlns=\"http://www.garmin.com/xmlschemas/ActivityExtension/v2\"><Watts>69</Watts></TPX></Extensions></Trackpoint><Trackpoint><Time>2008-03-03T23:09:34Z</Time><Position><LatitudeDegrees>35.860894</LatitudeDegrees><LongitudeDegrees>-78.893602</LongitudeDegrees></Position><AltitudeMeters>62.142</AltitudeMeters><DistanceMeters>13381.185</DistanceMeters><Cadence>95</Cadence><Extensions><TPX xmlns=\"http://www.garmin.com/xmlschemas/ActivityExtension/v2\"><Watts>84</Watts></TPX></Extensions></Trackpoint><Trackpoint><Time>2008-03-03T23:09:35Z</Time><Position><LatitudeDegrees>35.860916</LatitudeDegrees><LongitudeDegrees>-78.893748</LongitudeDegrees></Position><AltitudeMeters>61.662</AltitudeMeters><DistanceMeters>13394.587</DistanceMeters><Cadence>94</Cadence><Extensions><TPX xmlns=\"http://www.garmin.com/xmlschemas/ActivityExtension/v2\"><Watts>149</Watts></TPX></Extensions></Trackpoint><Trackpoint><Time>2008-03-03T23:09:36Z</Time><Position><LatitudeDegrees>35.860938</LatitudeDegrees><LongitudeDegrees>-78.893892</LongitudeDegrees></Position><AltitudeMeters>62.142</AltitudeMeters><DistanceMeters>13407.826</DistanceMeters><Cadence>94</Cadence><Extensions><TPX xmlns=\"http://www.garmin.com/xmlschemas/ActivityExtension/v2\"><Watts>148</Watts></TPX></Extensions></Trackpoint><Trackpoint><Time>2008-03-03T23:09:37Z</Time><Position><LatitudeDegrees>35.860960</LatitudeDegrees><LongitudeDegrees>-78.894034</LongitudeDegrees></Position><AltitudeMeters>62.142</AltitudeMeters><DistanceMeters>13420.849</DistanceMeters><Cadence>90</Cadence><Extensions><TPX xmlns=\"http://www.garmin.com/xmlschemas/ActivityExtension/v2\"><Watts>189</Watts></TPX></Extensions></Trackpoint><Trackpoint><Time>2008-03-03T23:09:38Z</Time><Position><LatitudeDegrees>35.860982</LatitudeDegrees><LongitudeDegrees>-78.894170</LongitudeDegrees></Position><AltitudeMeters>62.623</AltitudeMeters><DistanceMeters>13433.315</DistanceMeters><Cadence>88</Cadence><Extensions><TPX xmlns=\"http://www.garmin.com/xmlschemas/ActivityExtension/v2\"><Watts>159</Watts></TPX></Extensions></Trackpoint><Trackpoint><Time>2008-03-03T23:09:39Z</Time><Position><LatitudeDegrees>35.860999</LatitudeDegrees><LongitudeDegrees>-78.894301</LongitudeDegrees></Position><AltitudeMeters>63.584</AltitudeMeters><DistanceMeters>13445.208</DistanceMeters><Cadence>82</Cadence><Extensions><TPX xmlns=\"http://www.garmin.com/xmlschemas/ActivityExtension/v2\"><Watts>141</Watts></TPX></Extensions></Trackpoint><Trackpoint><Time>2008-03-03T23:09:40Z</Time><Position><LatitudeDegrees>35.861013</LatitudeDegrees><LongitudeDegrees>-78.894425</LongitudeDegrees></Position><AltitudeMeters>63.104</AltitudeMeters><DistanceMeters>13456.548</DistanceMeters><Cadence>80</Cadence><Extensions><TPX xmlns=\"http://www.garmin.com/xmlschemas/ActivityExtension/v2\"><Watts>182</Watts></TPX></Extensions></Trackpoint><Trackpoint><Time>2008-03-03T23:09:41Z</Time><Position><LatitudeDegrees>35.861022</LatitudeDegrees><LongitudeDegrees>-78.894545</LongitudeDegrees></Position><AltitudeMeters>63.104</AltitudeMeters><DistanceMeters>13467.396</DistanceMeters><Cadence>76</Cadence><Extensions><TPX xmlns=\"http://www.garmin.com/xmlschemas/ActivityExtension/v2\"><Watts>226</Watts></TPX></Extensions></Trackpoint><Trackpoint><Time>2008-03-03T23:09:42Z</Time><Position><LatitudeDegrees>35.861024</LatitudeDegrees><LongitudeDegrees>-78.894660</LongitudeDegrees></Position><AltitudeMeters>63.584</AltitudeMeters><DistanceMeters>13477.749</DistanceMeters><Cadence>72</Cadence><Extensions><TPX xmlns=\"http://www.garmin.com/xmlschemas/ActivityExtension/v2\"><Watts>235</Watts></TPX></Extensions></Trackpoint><Trackpoint><Time>2008-03-03T23:09:43Z</Time><Position><LatitudeDegrees>35.861022</LatitudeDegrees><LongitudeDegrees>-78.894771</LongitudeDegrees></Position><AltitudeMeters>64.065</AltitudeMeters><DistanceMeters>13487.723</DistanceMeters><Cadence>72</Cadence><Extensions><TPX xmlns=\"http://www.garmin.com/xmlschemas/ActivityExtension/v2\"><Watts>236</Watts></TPX></Extensions></Trackpoint><Trackpoint><Time>2008-03-03T23:09:44Z</Time><Position><LatitudeDegrees>35.861018</LatitudeDegrees><LongitudeDegrees>-78.894878</LongitudeDegrees></Position><AltitudeMeters>64.546</AltitudeMeters><DistanceMeters>13497.354</DistanceMeters><Cadence>78</Cadence><Extensions><TPX xmlns=\"http://www.garmin.com/xmlschemas/ActivityExtension/v2\"><Watts>196</Watts></TPX></Ex
